vi "Get LoopTunnel Terminals Names.vi"(8 "error in (no error)":errorcluster, 10 "Outer Terminal":refnum<vi>, 11 "Inside Terminals []":refnum<vi>[](array[refnum])) -> (0 "error out":errorcluster, 2 "Outer Terminal Wire Name":string, 3 "Inner Terminals Wires Names":string[](array[string]))   [LabVIEW 2014]
doc: "Returns array of names of connected wires to inner terminal (array) and outer terminal wire name (just one value)."
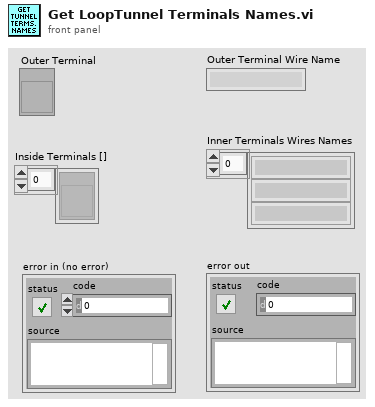
[diagram p1: front panel]
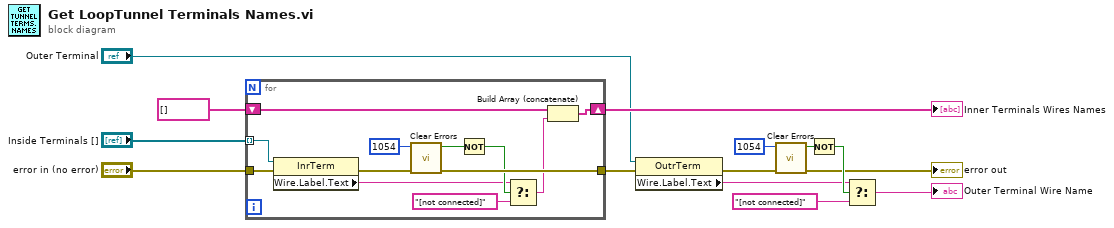
[diagram p0: block diagram]
diagram:
  n1 = for {
    tunnel: "Inside Terminals []" -> [w21] mode=indexing
    tunnel: "error in (no error)" -> [w22]
    tunnel: [w26] -> w10
    shift-right: [w17] -> w14
    shift-left: string[] [] -> [w15]
    n2 = property class="InrTerm"(reference=w21, error in=w22) -> (error out=w25:errorcluster, "Wire.Label.Text"=w19:string)  [unwired: 1 out]
    n3 = call <vilib>:"Clear Errors.vi"("error in (no error)"=w25, "specific error code to clear (0: all)"=1054) -> ("error out"=w26:errorcluster, "specific error cleared?"=w23:bool)  [unwired: 4 in]
    n4 = Not(x=w23) -> (.not. x?=w20:bool)
    n5 = Select(t=w19, s=w20, f="[not connected]") -> (s? t:f=w16:string)
    n6 = Build Array (concatenate)(w15, w16) -> (w17:string[])
  }
  "Inner Terminals Wires Names" <- w14
  n7 = property class="OutrTerm"(reference="Outer Terminal", error in=w10) -> (error out=w5:errorcluster, "Wire.Label.Text"=w3:string)  [unwired: 1 out]
  n8 = call <vilib>:"Clear Errors.vi"("error in (no error)"=w5, "specific error code to clear (0: all)"=1054) -> ("error out"=→"error out":errorcluster, "specific error cleared?"=w7:bool)  [unwired: 4 in]
  n9 = Not(x=w7) -> (.not. x?=w4:bool)
  n10 = Select(t=w3, s=w4, f="[not connected]") -> (s? t:f=→"Outer Terminal Wire Name":string)
